vi "Get Cursor Values.vi"(7 "error in (no error)":errorcluster, 10 "Waveform Graph Ref":refnum<vi>) -> (0 "error out":errorcluster, 1 "Cursor values":dbl[][](array[numeric]) format="%#_4p")   [LabVIEW 2019]
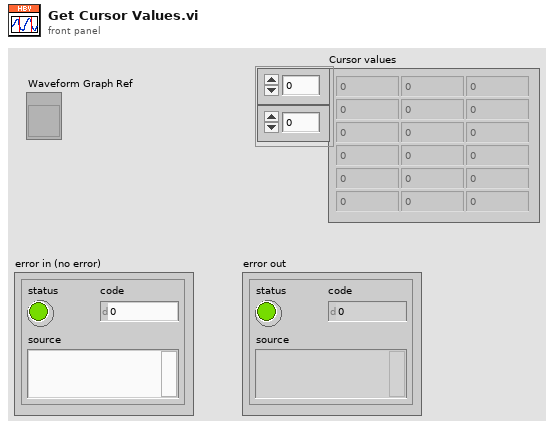
[diagram p1: front panel]
types:
  T1 = typedef "LVCursorListTypeDef.ctl" = cluster{"Name":string, "Color":u32, "Style":u8, "Point Style":u8, "Name Visible":bool, "Allow Drag":bool, "Cursor Mode":u32, "Plot":i32, "Index":i32, "Position":cluster{"X":dbl, "Y":dbl}, "X Scale":u32, "Y Scale":u32, "Watch Plots":i32[], "Watch All Plots":bool, "Plot Area":i32, "Label Offset":cluster{"X":dbl, "Y":dbl}}[]
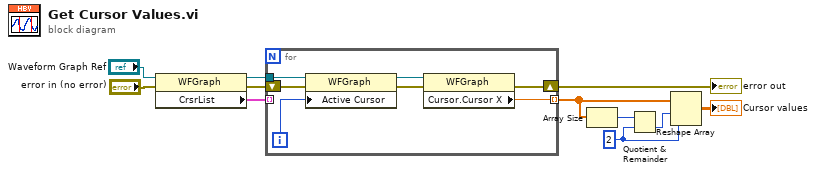
[diagram p0: block diagram]
diagram:
  w1 = 2
  n1 = property class="WFGraph"(reference="Waveform Graph Ref", error in="error in (no error)") -> (reference out=w6:refnum<vi>, error out=w11:errorcluster, "CrsrList"=w7:T1)
  n2 = for {
    tunnel: w7 -> [_] mode=indexing
    tunnel: [w12] -> w4 mode=indexing
    tunnel: w6 -> [w18]
    shift-right: [w13] -> w10
    shift-left: w11 -> [w16]
    i -> [w17]
    n3 = property class="WFGraph"(reference=w18, error in=w16, "Active Cursor"=w17) -> (reference out=w15:refnum<vi>, error out=w14:errorcluster)
    n4 = property class="WFGraph"(reference=w15, error in=w14) -> (error out=w13:errorcluster, "Cursor.Cursor X"=w12:dbl)  [unwired: 1 out]
  }
  "error out" <- w10
  n5 = Array Size(array=w4) -> (size(s)=w3:i32)
  n6 = Quotient & Remainder(x=w3, y=w1) -> (floor(x/y)=w2:i32)  [unwired: 1 out]
  n7 = Reshape Array(w4, w2, w1) -> (→"Cursor values":dbl[][])
